vi "4-7.vi"() -> (0 "次数":i32, 1 "随机数":i32, 2 "输入":i32)   [LabVIEW 2017]
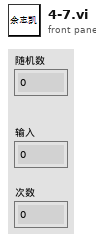
[diagram p1: front panel]
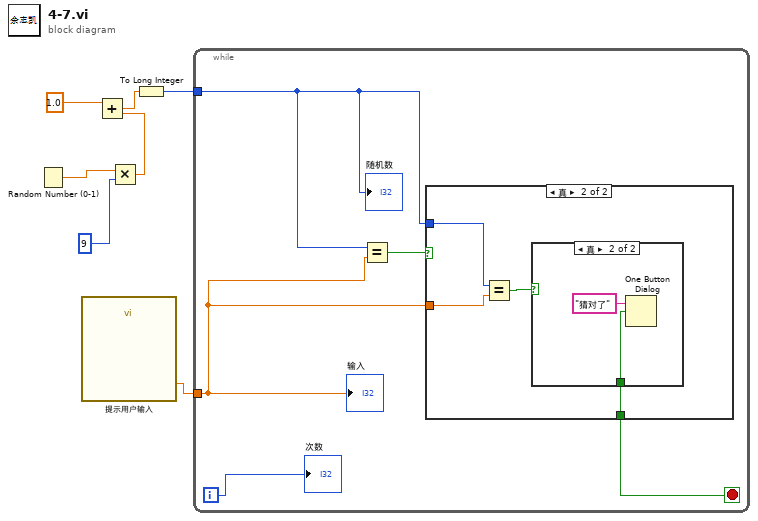
[diagram p0: block diagram]
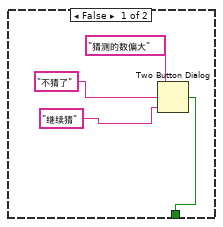
[diagram p2: hidden frame]
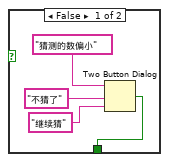
[diagram p3: hidden frame]
diagram:
  n1 = Random Number (0-1)() -> (number: 0 to 1=w4:dbl)
  n2 = call "提示用户输入"() -> ("请在1-1000猜"=w7:dbl)  [unwired: 17 in, 2 out]
  n3 = Multiply(x=w4, y=9) -> (x*y=w5:dbl)
  n4 = Add(x=1.0, y=w5) -> (x+y=w6:dbl)
  n5 = To Long Integer(number=w6) -> (32bit integer=w2:i32)
  n6 = while {
    tunnel: w7 -> [w10]
    tunnel: w2 -> [w8]
    i -> [w11]
    stop <- w12 stop-if-true
    n7 = Equal?(x=w8, y=w10) -> (x = y?=w9:bool)
    n8 = case shown="真" w9 {
      tunnel: w10 -> [_ w20]
      tunnel: w8 -> [_ w19]
      tunnel: [w15 w17] -> w12
      frame False {
        n9 = Two Button Dialog(message="猜测的数偏大", 1:"继续猜", 2:"不猜了") -> (T button?=w15:bool)
      }
      frame True {
        n10 = Equal?(x=w19, y=w20) -> (x = y?=w18:bool)
        n11 = case shown="真" w18 {
          tunnel: [w23 w25] -> w17
          frame False {
            n12 = Two Button Dialog(message="猜测的数偏小", 1:"继续猜", 2:"不猜了") -> (T button?=w23:bool)
          }
          frame True {
            n13 = One Button Dialog(message="猜对了" ("消息")) -> (true=w25:bool)  [unwired: 1 in]
          }
        }
      }
    }
    "次数" <- w11
    "输入" <- w10
    "随机数" <- w8
  }
